vi "index array (dbl with bool).vi"(4 "good":bool[](array[boolean]), 5 "array":dbl[](array[numeric])) -> (1 "indexed array":dbl[](array[numeric]))   [LabVIEW 2012, in "common.lvlib"]
uses:
  common.lvlib
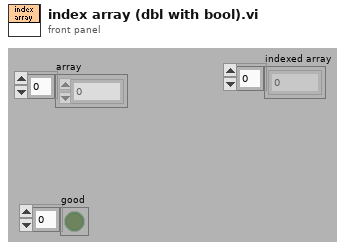
[diagram p1: front panel]
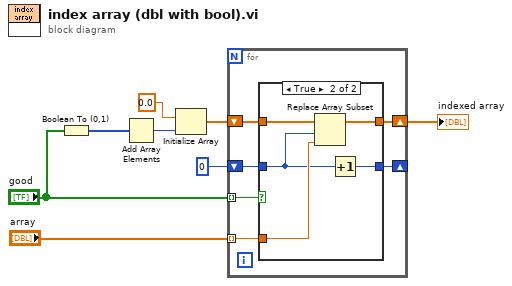
[diagram p0: block diagram]
diagram:
  n1 = Boolean To (0,1)(Boolean="good") -> (0, 1=w3:i16[])
  n2 = Add Array Elements(numeric array=w3) -> (sum=w8:i16)
  n3 = Initialize Array(0.0, w8) -> (w6:dbl[])
  n4 = for {
    tunnel: "good" -> [w14] mode=indexing
    tunnel: "array" -> [w11] mode=indexing
    shift-right: [w12] -> w4
    shift-left: w6 -> [w13]
    shift-right: [w9] -> _
    shift-left: 0 ("element") -> [w10]
    n5 = case shown="True" w14 {
      tunnel: w13 -> [w16 w21]
      tunnel: [w16 w20] -> w12
      tunnel: w11 -> [_ w19]
      tunnel: w10 -> [w15 w18]
      tunnel: [w15 w17] -> w9
      frame False {
      }
      frame True {
        n6 = Replace Array Subset(array=w21, new element=w19, index=w18) -> (w20:dbl[])
        n7 = Increment(x=w18) -> (x+1=w17:i32)
      }
    }
  }
  "indexed array" <- w4
